vi "计算圆与直线的焦点中心点.vi"(8 "error in (no error)":errorcluster caption="错误输入（无错误）", 9 "结束角度":dbl, 10 "起始角度":dbl, 11 "中心位置":T1={"Cent X"=277.0, "Cent Y"=190.0, "R"=190.0, "Color1Number"=20.0, "Color2Number"=50.0, "Color3Number"=40.0, "Color4Number"=70.0, "Color5Number"=90.0}) -> (0 "error out":errorcluster caption="错误输出", 3 "XY输出":cluster{"X":dbl, "Y":dbl})   [LabVIEW 2015]
panel:
  out "x*y 2":dbl
  out "sqrt(x) 2":dbl
  out "x-y 2":dbl
  out "x-y":dbl
  out "x/y":dbl
  out "tan(x)":dbl
  out "数字":u32
  # "0~90度=1\n90~180度=2\n180~270度=4\n270~360度=8"
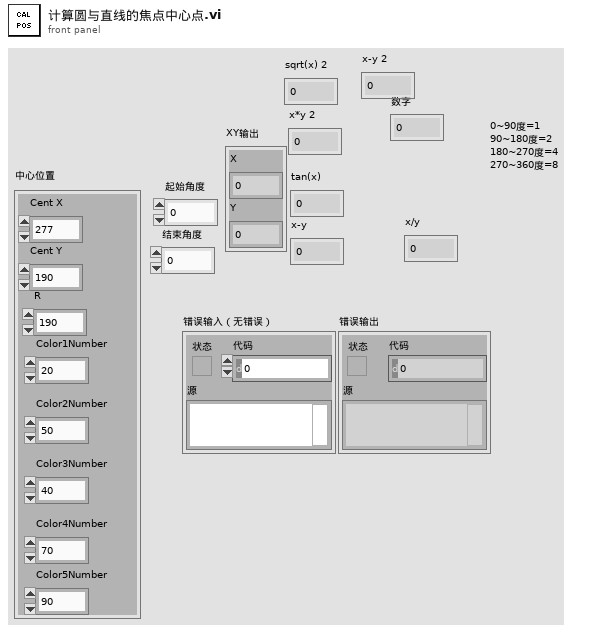
[diagram p1: front panel]
types:
  T1 = cluster{"Cent X":dbl, "Cent Y":dbl, "R":dbl, "Color1Number":dbl, "Color2Number":dbl, "Color3Number":dbl, "Color4Number":dbl, "Color5Number":dbl}
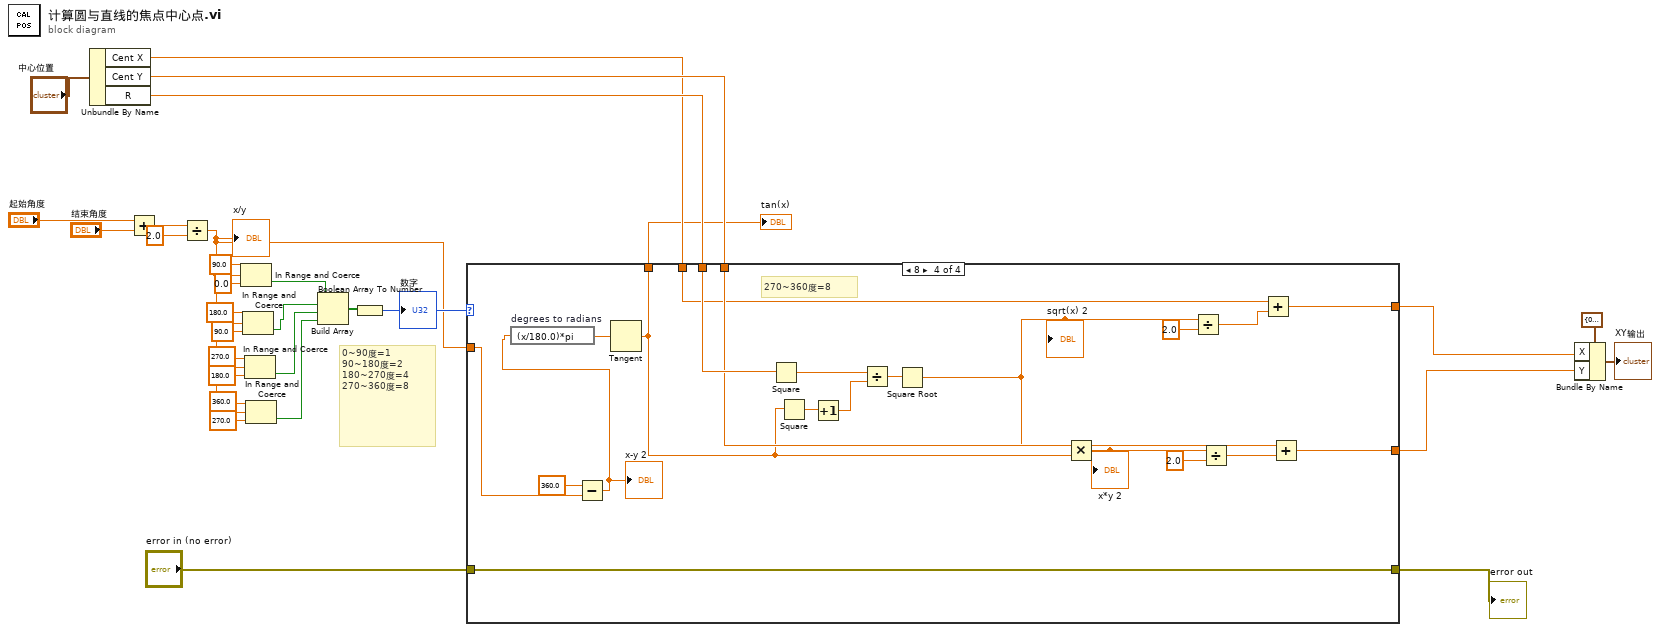
[diagram p0: block diagram]
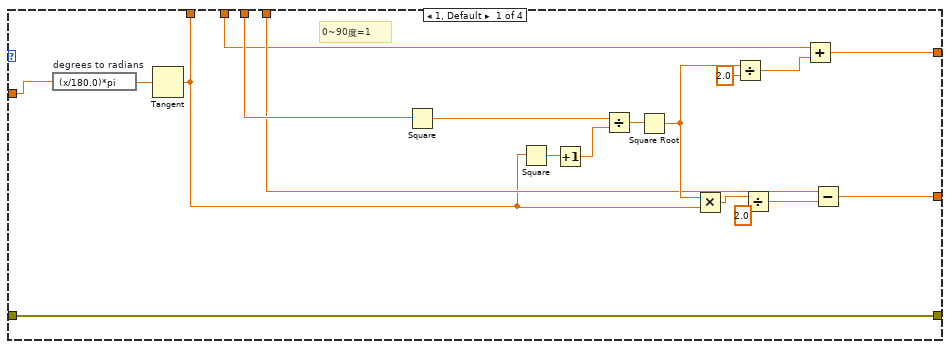
[diagram p2: hidden frame]
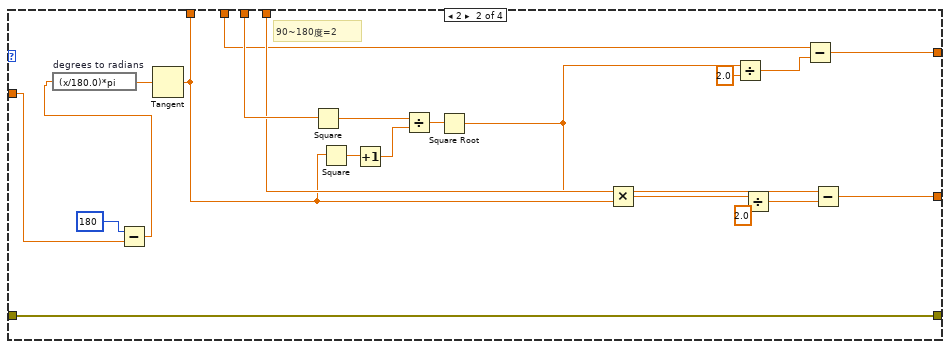
[diagram p3: hidden frame]
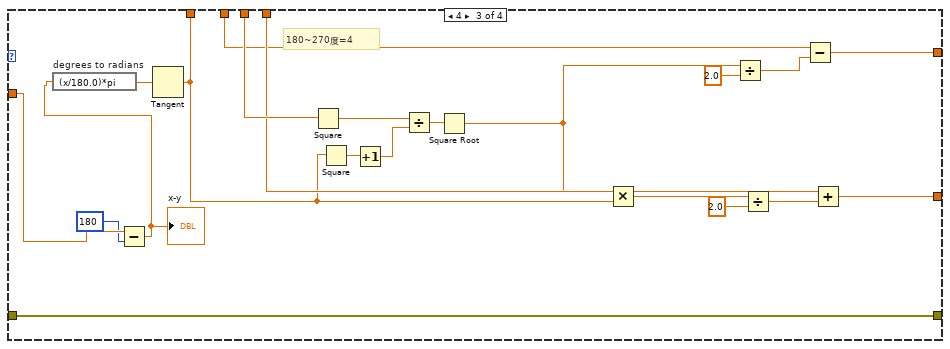
[diagram p4: hidden frame]
diagram:
  # "0~90度=1\n90~180度=2\n180~270度=4\n270~360度=8"
  n1 = Unbundle By Name("中心位置") -> ("Cent X"=w8:dbl, "Cent Y"=w9:dbl, "R"=w10:dbl)
  n2 = Add(x="起始角度", y="结束角度") -> (x+y=w28:dbl)
  n3 = Divide(x=w28, y=2.0) -> (x/y=w11:dbl)
  "x/y" <- w11
  n4 = In Range and Coerce(upper limit=90.0 ("上限"), x=w11, lower limit=0.0 ("下限")) -> (In Range?=w17:bool)  [unwired: 1 out]
  n5 = In Range and Coerce(upper limit=180.0 ("上限"), x=w11, lower limit=90.0 ("下限")) -> (In Range?=w16:bool)  [unwired: 1 out]
  n6 = In Range and Coerce(upper limit=270.0 ("上限"), x=w11, lower limit=180.0 ("下限")) -> (In Range?=w15:bool)  [unwired: 1 out]
  n7 = In Range and Coerce(upper limit=360.0 ("上限"), x=w11, lower limit=270.0 ("下限")) -> (In Range?=w14:bool)  [unwired: 1 out]
  n8 = Build Array(w17, w16, w15, w14) -> (w13:bool[])
  n9 = Boolean Array To Number(Boolean array=w13) -> (number=w12:u32)
  "数字" <- w12
  n10 = case shown="8" w12 {
    tunnel: w11 -> [w48 w53 w72 w93]
    tunnel: w10 -> [w37 w60 w81 w102]
    tunnel: w9 -> [w36 w59 w80 w101]
    tunnel: w8 -> [w35 w58 w79 w100]
    tunnel: [w34 w57 w78 w99] -> w5
    tunnel: [w33 w56 w77 w98] -> w4
    tunnel: [w32 w55 w76 w97] -> w7
    tunnel: "error in (no error)" -> [w31 w50 w73 w94]
    tunnel: [w31 w50 w73 w94] -> w1
    frame 1, Default {
      # "0~90度=1"
      n11 = expression code="(x/180.0)*pi" "degrees to radians"(w48) -> (w49:dbl)
      n12 = Tangent(1:w49) -> (0:w32:dbl)
      n13 = Square(x=w37) -> (x^2=w39:dbl)
      n14 = Square(x=w32) -> (x^2=w38:dbl)
      n15 = Increment(x=w38) -> (x+1=w40:dbl)
      n16 = Divide(x=w39, y=w40) -> (x/y=w41:dbl)
      n17 = Square Root(x=w41) -> (sqrt(x)=w43:dbl)
      n18 = Multiply(x=w43, y=w32) -> (x*y=w45:dbl)
      n19 = Divide(x=w43, y=2.0) -> (x/y=w44:dbl)
      n20 = Divide(x=w45, y=2.0) -> (x/y=w47:dbl)
      n21 = Add(x=w35, y=w44) -> (x+y=w34:dbl)
      n22 = Subtract(x=w36, y=w47) -> (x-y=w33:dbl)
    }
    frame 2 {
      # "90~180度=2"
      n23 = Subtract(x=180, y=w53) -> (x-y=w52:dbl)
      n24 = expression code="(x/180.0)*pi" "degrees to radians"(w52) -> (w70:dbl)
      n25 = Tangent(1:w70) -> (0:w55:dbl)
      n26 = Square(x=w60) -> (x^2=w62:dbl)
      n27 = Square(x=w55) -> (x^2=w61:dbl)
      n28 = Increment(x=w61) -> (x+1=w63:dbl)
      n29 = Divide(x=w62, y=w63) -> (x/y=w64:dbl)
      n30 = Square Root(x=w64) -> (sqrt(x)=w51:dbl)
      n31 = Multiply(x=w51, y=w55) -> (x*y=w67:dbl)
      n32 = Divide(x=w51, y=2.0) -> (x/y=w66:dbl)
      n33 = Divide(x=w67, y=2.0) -> (x/y=w69:dbl)
      n34 = Subtract(x=w58, y=w66) -> (x-y=w57:dbl)
      n35 = Subtract(x=w59, y=w69) -> (x-y=w56:dbl)
    }
    frame 4 {
      # "180~270度=4"
      n36 = Subtract(x=w72, y=180) -> (x-y=w75:dbl)
      "x-y" <- w75
      n37 = expression code="(x/180.0)*pi" "degrees to radians"(w75) -> (w91:dbl)
      n38 = Tangent(1:w91) -> (0:w76:dbl)
      n39 = Square(x=w81) -> (x^2=w83:dbl)
      n40 = Square(x=w76) -> (x^2=w82:dbl)
      n41 = Increment(x=w82) -> (x+1=w84:dbl)
      n42 = Divide(x=w83, y=w84) -> (x/y=w85:dbl)
      n43 = Square Root(x=w85) -> (sqrt(x)=w74:dbl)
      n44 = Multiply(x=w74, y=w76) -> (x*y=w88:dbl)
      n45 = Divide(x=w74, y=2.0) -> (x/y=w87:dbl)
      n46 = Divide(x=w88, y=2.0) -> (x/y=w90:dbl)
      n47 = Subtract(x=w79, y=w87) -> (x-y=w78:dbl)
      n48 = Add(x=w80, y=w90) -> (x+y=w77:dbl)
    }
    frame 8 {
      # "270~360度=8"
      n49 = Subtract(x=360.0, y=w93) -> (x-y=w96:dbl)
      "x-y 2" <- w96
      n50 = expression code="(x/180.0)*pi" "degrees to radians"(w96) -> (w112:dbl)
      n51 = Tangent(1:w112) -> (0:w97:dbl)
      n52 = Square(x=w102) -> (x^2=w104:dbl)
      n53 = Square(x=w97) -> (x^2=w103:dbl)
      n54 = Increment(x=w103) -> (x+1=w105:dbl)
      n55 = Divide(x=w104, y=w105) -> (x/y=w106:dbl)
      n56 = Square Root(x=w106) -> (sqrt(x)=w95:dbl)
      "sqrt(x) 2" <- w95
      n57 = Multiply(x=w95, y=w97) -> (x*y=w109:dbl)
      "x*y 2" <- w109
      n58 = Divide(x=w95, y=2.0) -> (x/y=w108:dbl)
      n59 = Divide(x=w109, y=2.0) -> (x/y=w111:dbl)
      n60 = Add(x=w100, y=w108) -> (x+y=w99:dbl)
      n61 = Add(x=w101, y=w111) -> (x+y=w98:dbl)
    }
  }
  "tan(x)" <- w7
  "error out" <- w1
  n62 = Bundle By Name(cluster=cluster{"X":dbl, "Y":dbl} {"X"=0.0, "Y"=0.0} ("输入簇"), "X"=w5, "Y"=w4) -> (→"XY输出":cluster{"X":dbl, "Y":dbl})
